vi "Autonomous Independent.vi"   [LabVIEW 2019]
doc: "This VI is called when autonomous begins, and will automatically be terminated when autonomous ends. You can carry out timed or sensor driven robot movement independently without needing to return to the caller."
uses:
  Motion_Profiler_Class-master/MotionProfiles.lvclass
  <vilib>/Rock Robotics/WPI/Solenoid/WPI_SolenoidValue.ctl
  <vilib>/Rock Robotics/WPI/ThirdParty/Phoenix-LabVIEW/Motor Controller/Sensor/CTRE_Phoenix_MotorControl_SetIntegratedSensorPosition_TalonFX.vi
  <vilib>/Rock Robotics/Network Tables/NT Write Variant.vi
  <vilib>/Rock Robotics/WPI/Solenoid/WPI_SolenoidSetEnum.vi
  <vilib>/Rock Robotics/Network Tables/NT Read String.vi
  <vilib>/Utility/file.llb/Read Delimited Spreadsheet (string).vi
  <vilib>/Utility/file.llb/Read Delimited Spreadsheet (DBL).vi
  <vilib>/Rock Robotics/Network Tables/NT Write Number.vi
panel:
  # "Be sure to right-click and choose Data Operations>>Make Current Value default if you want to save the array values with the VI"
types:
  T1 = typedef "WPI_SolenoidValue.ctl" = enum16{"Off", "On", "Forward", "Reverse"}
  T2 = typedef "WPI_MotorControlDeviceRef.ctl" = cluster{"DeviceStatus":errorcluster, "Type":T3, "PWM":cluster{"PWM Channel":T4, "DeadBand":T5}, "CAN":cluster{"Device Number":u8, "SetOutput VI Ref":variant, "GetOutput VI Ref":variant, "Enable VI Ref":variant, "Disable VI Ref":variant, "Data":variant}, "Invert":bool, "DIO PWM":cluster{"PWM \"Enable\" Channel":T4, "DIOChannel":T6, "PWM Rate":dbl}}
  T3 = typedef "WPI_MotorControlType.ctl" = enum16{"PWM", "CAN", "DIO PWM"}
  T4 = typedef "FPGA_DIOPWMChannel.ctl" = enum8{"PWM 0", "PWM 1", "PWM 2", "PWM 3", "PWM 4", "PWM 5", "PWM 6", "PWM 7", "PWM 8", "PWM 9", "PWM MXP 0", "PWM MXP 1", "PWM MXP 2", "PWM MXP 3", "PWM MXP 4", "PWM MXP 5", "PWM MXP 6", "PWM MXP 7", "PWM MXP 8", "PWM MXP 9", "Invalid"}
  T5 = typedef "WPI_PWMDeadband.ctl" = cluster{"Name":string, "maxPositivePwm":i32, "minPositivePwm":i32, "centerPwm":i32, "maxNegativePwm":i32, "minNegativePwm":i32, "angularRange":u16}
  T6 = typedef "FPGA_DIOChannel.ctl" = enum8{"DIO 0", "DIO 1", "DIO 2", "DIO 3", "DIO 4", "DIO 5", "DIO 6", "DIO 7", "DIO 8", "DIO 9", "DIO MXP 0", "DIO MXP 1", "DIO MXP 2", "DIO MXP 3", "DIO MXP 4", "DIO MXP 5", "DIO MXP 6", "DIO MXP 7", "DIO MXP 8", "DIO MXP 9", "DIO MXP 10", "DIO MXP 11", "DIO MXP 12", "DIO MXP 13", "DIO MXP 14", "DIO MXP 15", "SPI Port CS1", "SPI Port CS2", "SPI Port CS3", "SPI Port MISO", "SPI Port MOSI", "Invalid"}
  T7 = typedef "WPI_SolenoidDevRef.ctl" = cluster{"DevStatus":errorcluster, "Pneumatics Control Module":u8, "Forward Solenoid Channel":T8, "Reverse Solenoid Channel":T8}
  T8 = typedef "WPI_SolenoidChannel.ctl" = enum8{"Solenoid 0", "Solenoid 1", "Solenoid 2", "Solenoid 3", "Solenoid 4", "Solenoid 5", "Solenoid 6", "Solenoid 7", "Invalid"}
  T9 = typedef "MotionProfiles.lvclass/MotionProfile_MP_Class_Status.ctl" = cluster{"Motion Profile Status":cluster{"Top Buffer Remaining":i32, "Top Buffer Count":i32, "Bottom Buffer Count":i32, "Has Underrun?":bool, "Is Underrun?":bool, "Active Point Valid?":bool, "Is Last?":bool, "Profile Slot Select 0":i32, "Output Enable":i32, "Time Duration (ms)":i32, "Profile Slot Select 1":i32}, "TalonState":T10, "MP Is Done":bool, "MP Is Executing":bool, "Set_Vel_(u/100ms)":i32, "Set_Pos_(u)":i32, "Act_Vel_(u/100ms)":i32, "Act_Pos(u)":i32, "Throtle":dbl}
  T10 = typedef "MotionProfiles.lvclass/MotionProfile_TalonSetValueEnum.ctl" = enum16{"Disable", "Enable", "Hold"}
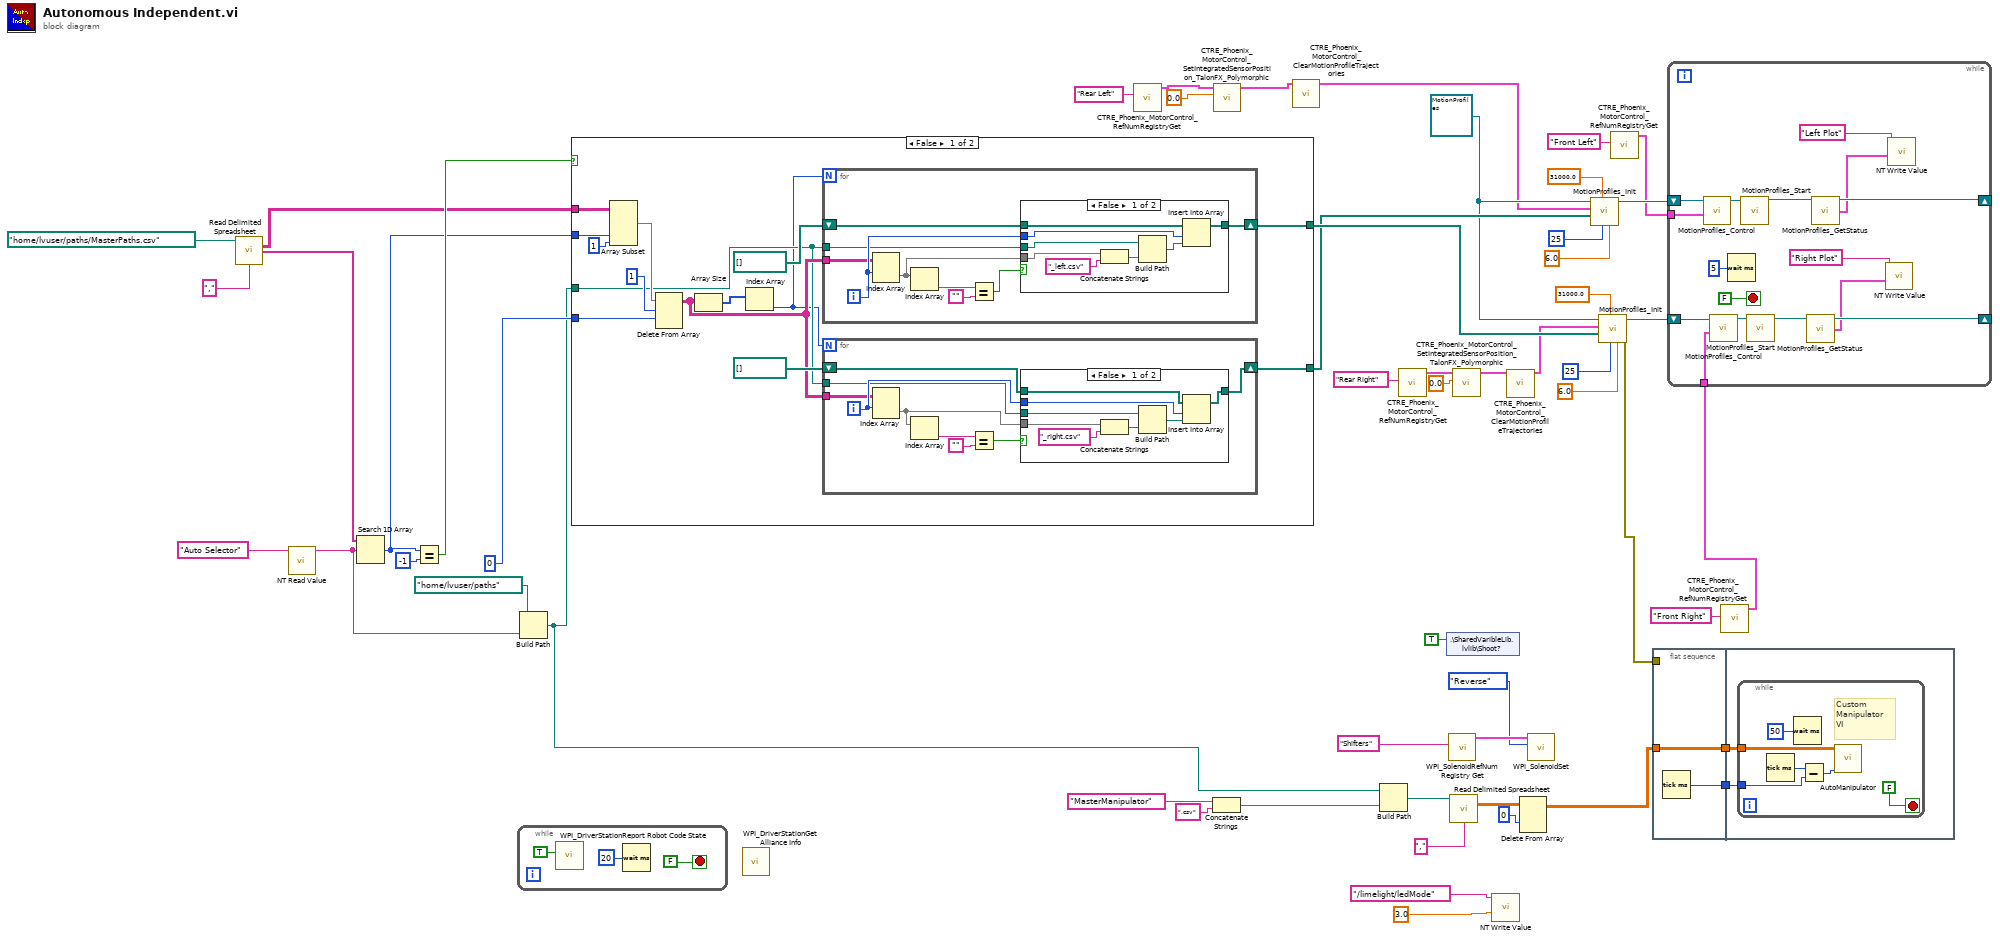
[diagram p0: block diagram]
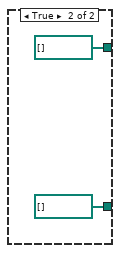
[diagram p4: hidden frame]
diagram:
  w30 = refnum<class "MotionProfiles.lvclass"> refnum ("MotionProfiles.lvclass")
  n1 = call-poly <vilib>:"Read Delimited Spreadsheet.vi"("file path (dialog if empty)"=path "/home/lvuser/paths/MasterPaths.csv" ("file path (use dialog)"), "delimiter (\\t)"="," ("delimiter (\\t)")) -> ("all rows"=w41:string[][], "first row"=w44:string[])  [unwired: 8 in, 4 out]
  n2 = call-poly <vilib>:"NT Read Value.vi"("Name"="Auto Selector") -> ("String"=w15:string)  [unwired: 9 in, 1 out]
  n3 = Search 1D Array(1D array=w44, element=w15) -> (index of element=w40:i32)  [unwired: 1 in]
  n4 = Equal?(x=w40, y=-1) -> (x = y?=w42:bool)
  n5 = while {
    stop <- FALSE stop-if-true
    n6 = call <vilib>:"WPI_DriverStationReport Robot Code State.vi"("Autonomous"=TRUE) -> ()  [unwired: 10 in, 1 out]
    n7 = Wait (ms)(milliseconds to wait=u32 20) -> ()  [unwired: 1 out]
  }
  n8 = Build Path(base path=path "/home/lvuser/paths" ("file path (use dialog)"), name or relative path=w15) -> (appended path=w12:path)
  n9 = case shown="False" w42 {
    tunnel: w41 -> [w71 _]
    tunnel: w40 -> [w63 _]
    tunnel: [w59 path[] [] ("CSV File Path")] -> w35
    tunnel: [w65 path[] [] ("CSV File Path")] -> w31
    tunnel: w12 -> [w60 _]
    tunnel: 0 ("index (row)") -> [w64 _]
    frame False {
      n10 = Array Subset(array=w71, index (col)=w63, length (col)=1 ("length")) -> (w69:string[][])  [unwired: 2 in]
      n11 = Delete From Array(array=w69, length=1, index (row)=w64) -> (array with subset deleted=w61:string[][])  [unwired: 1 in, 1 out]
      n12 = Array Size(array=w61) -> (size(s)=w67:i32[])
      n13 = Index Array(array=w67) -> (element=w58:i32)  [unwired: 1 in]
      n14 = for {
        N: w58 -> [_]
        shift-right: [w79] -> w59
        shift-left: path[] [] ("CSV File Path") -> [w80]
        tunnel: w61 -> [w77]
        tunnel: w60 -> [w72]
        i -> [w78]
        n15 = Index Array(array=w77, index (row)=w78) -> (element=w74:string[])  [unwired: 1 in]
        n16 = Index Array(array=w74) -> (element=w73:string)  [unwired: 1 in]
        n17 = Equal?(x=w73, y="") -> (x = y?=w76:bool)
        n18 = case shown="False" w76 {
          tunnel: w80 -> [w88 w89]
          tunnel: [w87 w89] -> w79
          tunnel: w78 -> [w86 _]
          tunnel: w74 -> [w85 _]
          tunnel: w72 -> [w81 _]
          frame False {
            n19 = Concatenate Strings(w85, "_left.csv" ("string")) -> (w83:string)
            n20 = Build Path(base path=w81, name or relative path=w83) -> (appended path=w82:path)
            n21 = Insert Into Array(array=w88, index=w86, new element=w82) -> (w87:path[])
          }
          frame True {
          }
        }
      }
      n22 = for {
        N: w58 -> [_]
        shift-right: [w97] -> w65
        shift-left: path[] [] ("CSV File Path") -> [w98]
        tunnel: w61 -> [w95]
        tunnel: w60 -> [w94]
        i -> [w96]
        n23 = Index Array(array=w95, index (row)=w96) -> (element=w91:string[])  [unwired: 1 in]
        n24 = Index Array(array=w91) -> (element=w90:string)  [unwired: 1 in]
        n25 = Equal?(x=w90, y="") -> (x = y?=w93:bool)
        n26 = case shown="False" w93 {
          tunnel: w98 -> [w106 w107]
          tunnel: [w105 w107] -> w97
          tunnel: w96 -> [w104 _]
          tunnel: w91 -> [w103 _]
          tunnel: w94 -> [w99 _]
          frame False {
            n27 = Concatenate Strings(w103, "_right.csv" ("string")) -> (w101:string)
            n28 = Build Path(base path=w99, name or relative path=w101) -> (appended path=w100:path)
            n29 = Insert Into Array(array=w106, index=w104, new element=w100) -> (w105:path[])
          }
          frame True {
          }
        }
      }
    }
    frame True {
    }
  }
  n30 = call <vilib>:"WPI_DriverStationGet Alliance Info.vi"() -> ()  [unwired: 12 out]
  n31 = call <vilib>:"CTRE_Phoenix_MotorControl_RefNumRegistryGet.vi"("refnum name"="Rear Left") -> ("PhoenixMotorControlDevRef"=w49:T2)  [unwired: 9 in, 1 out]
  n32 = Concatenate Strings("MasterManipulator" ("string"), ".csv" ("string")) -> (w24:string)
  n33 = call-poly <vilib>:"CTRE_Phoenix_MotorControl_SetIntegratedSensorPosition_TalonFX_Polymorphic.vi"("New Position"=0.0, "PhoenixMotorControlDevRef"=w49) -> ("PhoenixMotorControlDevRef"=w2:T2)  [unwired: 8 in, 1 out]
  n34 = call <vilib>:"CTRE_Phoenix_MotorControl_ClearMotionProfileTrajectories.vi"("PhoenixMotorControlDevRef"=w2) -> ("PhoenixMotorControlDevRef"=w1:T2)  [unwired: 13 in, 1 out]
  n35 = Build Path(base path=w12, name or relative path=w24) -> (appended path=w22:path)
  n36 = call <vilib>:"CTRE_Phoenix_MotorControl_RefNumRegistryGet.vi"("refnum name"="Rear Right") -> ("PhoenixMotorControlDevRef"=w47:T2)  [unwired: 9 in, 1 out]
  n37 = shared-variable ".\\SharedVaribleLib.lvlib\\Shoot?"(TRUE ("Shoot?")) -> ()  [unwired: 1 in, 1 out]
  n38 = call <vilib>:"WPI_SolenoidRefNum Registry Get.vi"("refnum name"="Shifters") -> ("SolenoidDevRef"=w9:T7)  [unwired: 9 in, 1 out]
  n39 = call-poly <vilib>:"Read Delimited Spreadsheet.vi"("file path (dialog if empty)"=w22, "delimiter (\\t)"="," ("delimiter (\\t)")) -> ("all rows"=w25:dbl[][])  [unwired: 8 in, 5 out]
  n40 = call-poly <vilib>:"CTRE_Phoenix_MotorControl_SetIntegratedSensorPosition_TalonFX_Polymorphic.vi"("New Position"=0.0, "PhoenixMotorControlDevRef"=w47) -> ("PhoenixMotorControlDevRef"=w4:T2)  [unwired: 8 in, 1 out]
  n41 = call-poly <vilib>:"NT Write Value.vi"("Numeric"=3.0 ("Default Value"), "Name"="/limelight/ledMode") -> ()  [unwired: 9 in, 1 out]
  n42 = call <vilib>:"CTRE_Phoenix_MotorControl_ClearMotionProfileTrajectories.vi"("PhoenixMotorControlDevRef"=w4) -> ("PhoenixMotorControlDevRef"=w3:T2)  [unwired: 13 in, 1 out]
  n43 = Delete From Array(array=w25, index (row)=0) -> (array with subset deleted=w21:dbl[][])  [unwired: 2 in, 1 out]
  n44 = call-poly <vilib>:"WPI_SolenoidSet.vi"("Value"=WPI_SolenoidValue."Reverse", "SolenoidDevRef"=w9) -> ()  [unwired: 8 in, 2 out]
  n45 = call "MotionProfiles_Init.vi"("Wheel_Diameter (in)"=6.0, "MP_Frame_Rate_(ms)"=25, "Encoder_CPR_4x"=31000.0, "CSV File Path"=w31, "PhoenixMotorControlDevRef"=w1, "MotionProfiles in"=w30) -> ("MotionProfiles out"=w18:refnum<class "MotionProfiles.lvclass">)  [unwired: 4 in, 1 out]
  n46 = call "MotionProfiles_Init.vi"("Wheel_Diameter (in)"=6.0, "MP_Frame_Rate_(ms)"=25, "Encoder_CPR_4x"=31000.0, "CSV File Path"=w35, "PhoenixMotorControlDevRef"=w3, "MotionProfiles in"=w30) -> ("error out"=w20:errorcluster, "MotionProfiles out"=w19:refnum<class "MotionProfiles.lvclass">)  [unwired: 4 in]
  n47 = call <vilib>:"CTRE_Phoenix_MotorControl_RefNumRegistryGet.vi"("refnum name"="Front Left") -> ("PhoenixMotorControlDevRef"=w17:T2)  [unwired: 9 in, 1 out]
  n48 = flat-sequence {
    tunnel: [w111] -> w29
    tunnel: w21 -> [w110]
    tunnel: [w110] -> w28
    tunnel: w20 -> [_]
    tunnel: w29 -> [w113]
    tunnel: w28 -> [w112]
    frame #0 {
      n49 = Tick Count (ms)() -> (millisecond timer value=w111:u32)
    }
    frame #1 {
      n50 = while {
        tunnel: w113 -> [w117]
        tunnel: w112 -> [w114]
        stop <- FALSE stop-if-true
        # "Custom\nManipulator\nVI"
        n51 = Tick Count (ms)() -> (millisecond timer value=w118:u32)
        n52 = Wait (ms)(milliseconds to wait=u32 50) -> ()  [unwired: 1 out]
        n53 = Subtract(x=w118, y=w117) -> (x-y=w115:u32)
        n54 = call "AutoManipulator.vi"("Time"=w115, "array"=w114) -> ()  [unwired: 10 in]
      }
    }
  }
  n55 = call <vilib>:"CTRE_Phoenix_MotorControl_RefNumRegistryGet.vi"("refnum name"="Front Right") -> ("PhoenixMotorControlDevRef"=w16:T2)  [unwired: 9 in, 1 out]
  n56 = while {
    shift-right: [w124] -> _
    shift-left: w19 -> [w131]
    shift-right: [w125] -> _
    shift-left: w18 -> [w130]
    tunnel: w17 -> [w129]
    tunnel: w16 -> [w128]
    stop <- FALSE stop-if-true
    n57 = call "MotionProfiles_Control.vi"("PhoenixMotorControlDevRef Slave"=w129, "MotionProfiles in"=w130) -> ("MotionProfiles out"=w132:refnum<class "MotionProfiles.lvclass">)  [unwired: 8 in, 1 out]
    n58 = call "MotionProfiles_Control.vi"("PhoenixMotorControlDevRef Slave"=w128, "MotionProfiles in"=w131) -> ("MotionProfiles out"=w133:refnum<class "MotionProfiles.lvclass">)  [unwired: 8 in, 1 out]
    n59 = Wait (ms)(milliseconds to wait=u32 5) -> ()  [unwired: 1 out]
    n60 = call "MotionProfiles_Start.vi"("MotionProfiles in"=w132) -> ("MotionProfiles out"=w126:refnum<class "MotionProfiles.lvclass">)  [unwired: 9 in, 1 out]
    n61 = call "MotionProfiles_Start.vi"("MotionProfiles in"=w133) -> ("MotionProfiles out"=w127:refnum<class "MotionProfiles.lvclass">)  [unwired: 9 in, 1 out]
    n62 = call "MotionProfiles_GetStatus.vi"("MotionProfiles in"=w127) -> ("MotionProfiles out"=w124:refnum<class "MotionProfiles.lvclass">, "MP_Class_Status"=w123:T9)  [unwired: 12 in, 1 out]
    n63 = call "MotionProfiles_GetStatus.vi"("MotionProfiles in"=w126) -> ("MotionProfiles out"=w125:refnum<class "MotionProfiles.lvclass">, "MP_Class_Status"=w120:T9)  [unwired: 12 in, 1 out]
    n64 = call-poly <vilib>:"NT Write Value.vi"("Variant"=w123, "Name"="Right Plot") -> ()  [unwired: 9 in, 1 out]
    n65 = call-poly <vilib>:"NT Write Value.vi"("Variant"=w120, "Name"="Left Plot") -> ()  [unwired: 9 in, 1 out]
  }
